vi "ReadOffsetGainVals.vi"(8 "error in":errorcluster) -> (0 "error out":errorcluster, 3 "Array":dbl[](array[numeric]))   [LabVIEW 2023, in "QSM - IODocs.lvlib"]
uses:
  QSM - IODocs.lvlib
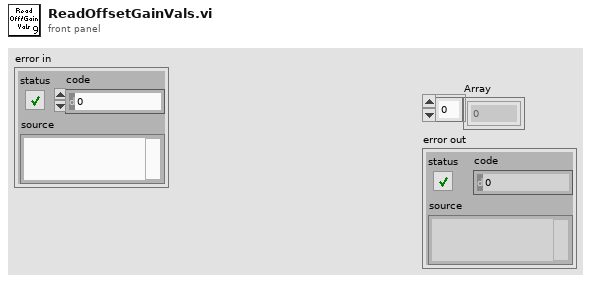
[diagram p1: front panel]
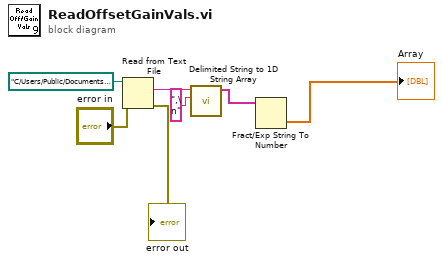
[diagram p0: block diagram]
diagram:
  n1 = Read from Text File(file (use dialog)=path "C:/Users/Public/Documents/Grid2093/IO/OffsetGain.txt", error in="error in") -> (text=w6:string, error out=→"error out":errorcluster)  [unwired: 2 in, 2 out]
  n2 = call <vilib>:"Delimited String to 1D String Array.vi"("delimiter"=",\n", "delimited string"=w6) -> ("string array"=w4:string[])  [unwired: 9 in]
  n3 = Fract/Exp String To Number(string=w4) -> (number=→"Array":dbl[])  [unwired: 3 in, 1 out]
